vi "P4CMD Open Project.vi"(8 "error in (no error)":errorcluster, 11 "configuration data":string) -> (0 "error out":errorcluster, 2 "status message":string, 3 "source control reference out":T1)   [LabVIEW 2017, in "NI_SCC_P4CMD.lvlib"]
uses:
  <vilib>/SourceControl/Providers/P4CMD/NI_SCC_P4CMD.lvlib
  <vilib>/SourceControl/sccapi/SCCAPI Refnum.ctl
  <vilib>/SourceControl/Providers/P4CMD/P4CMD Mgr Functions.ctl
  <vilib>/SourceControl/support/SCCSup Message Strings GLBL.vi
  <vilib>/SourceControl/sccapi/NI_SCC.lvlib
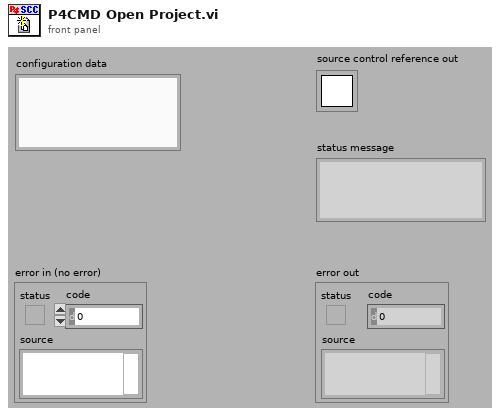
[diagram p1: front panel]
types:
  T1 = typedef "NI_SCC.lvlib/SCCAPI Refnum.ctl" = refnum<k1>
  T2 = typedef "NI_SCC_P4CMD.lvlib/P4CMD Mgr Functions.ctl" = enum16{"Init", "Open", "Set Config Opts", "Initialized?", "IsRefValid?", "Get Config Opts", "Get Global Commands", "Close", "Uninit"}
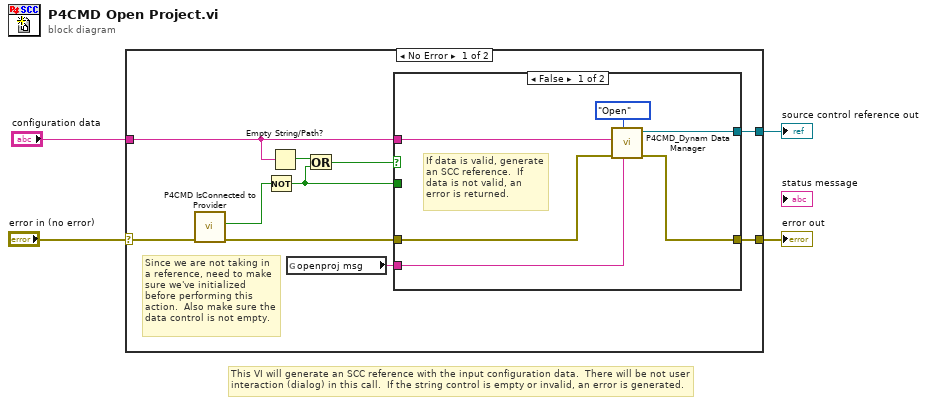
[diagram p0: block diagram]
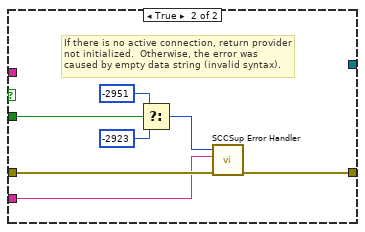
[diagram p2: hidden frame]
diagram:
  # "This VI will generate an SCC reference with the input configuration data.  There will be not user interaction (dialog) in this call.  If the string control is empty or invalid, an error is generated."
  n1 = case shown="No Error" "error in (no error)" {
    selector: "error in (no error)" -> [w11 w28]
    tunnel: [w14 _] -> w2
    tunnel: [w6 w28] -> w3
    tunnel: "configuration data" -> [w13 _]
    frame No Error {
      # "Since we are not taking in a reference, need to make sure we've initialized before performing this action.  Also make sure the data control is not empty."
      n2 = call <vilib>:"P4CMD IsConnected to Provider.vi"("error in (no error)"=w11) -> ("error out"=w7:errorcluster, "active connection?"=w9:bool)  [unwired: 9 in]
      n3 = Not(x=w9) -> (.not. x?=w8:bool)
      n4 = Empty String/Path?(string/path=w13) -> (empty?=w12:bool)
      n5 = global read "SCCSup Message Strings GLBL.vi" "openproj msg"() -> (w5:string)
      n6 = Or(x=w12, y=w8) -> (x .or. y?=w10:bool)
      n7 = case shown="False" w10 {
        tunnel: [w17 _] -> w14
        tunnel: w13 -> [w20 _]
        tunnel: w8 -> [_ w27]
        tunnel: w7 -> [w18 w23]
        tunnel: [w16 w22] -> w6
        tunnel: w5 -> [w15 w21]
        frame False {
          # "If data is valid, generate an SCC reference.  If data is not valid, an error is returned."
          n8 = call <vilib>:"P4CMD_Dynam Data Manager.vi"("operation message"=w15, "function"=P4CMD_Mgr_Functions."Open", "error in (no error)"=w18, "configuration data"=w20) -> ("error out"=w16:errorcluster, "source control reference out"=w17:T1)  [unwired: 2 in, 4 out]
        }
        frame True {
          # "If there is no active connection, return provider not initialized.  Otherwise, the error was caused by empty data string (invalid syntax)."
          n9 = Select(t=-2951 ("result"), s=w27, f=-2923 ("result")) -> (s? t:f=w24:i32)
          n10 = call <vilib>:"SCCSup Error Handler.vi"("error in (no error)"=w23, "operation message"=w21, "scc error code"=w24) -> ("error out"=w22:errorcluster)  [unwired: 8 in]
        }
      }
    }
    frame Error {
    }
  }
  "error out" <- w3
  "source control reference out" <- w2
